vi "Lab0_labview_front_panel.vi"() -> ()   [LabVIEW 2020]
panel:
  in  "Simulation Length":dbl=40.0
  out "Steady state value reached":bool=TRUE
  out "Waveform Chart":dbl(graph)=0.4999988027378587
  out "Current y_n":dbl
  in  "delta t":dbl=0.1
  out "Current Simulation step n":i32
  in  "Stop Simulation":bool
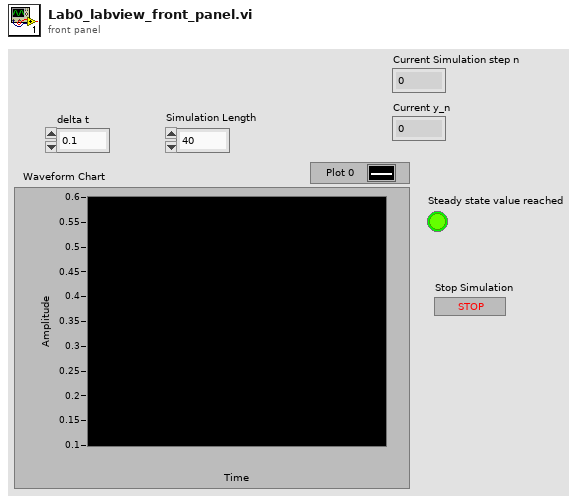
[diagram p1: front panel]
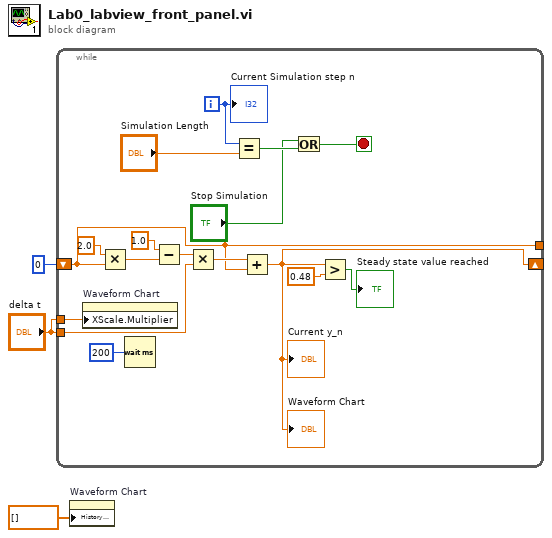
[diagram p0: block diagram]
diagram:
  n1 = while {
    shift-right: [w11] -> _
    shift-left: 0 -> [w10]
    tunnel: "delta t" -> [w15]
    tunnel: [w10] -> _
    tunnel: "delta t" -> [w4]
    i -> [w5]
    stop <- w7 stop-if-true
    n2 = property on="Waveform Chart" class="WFChart (strict)"("XScale.Multiplier"=w4) -> ()  [unwired: 2 in, 2 out]
    n3 = Multiply(x=2.0, y=w10) -> (x*y=w18:dbl)
    n4 = Wait (ms)(milliseconds to wait=u32 200) -> ()  [unwired: 1 out]
    n5 = Subtract(x=1.0, y=w18) -> (x-y=w16:dbl)
    n6 = Multiply(x=w16, y=w15) -> (x*y=w14:dbl)
    n7 = Equal?(x=w5, y="Simulation Length") -> (x = y?=w9:bool)
    n8 = Add(x=w14, y=w10) -> (x+y=w11:dbl)
    "Waveform Chart" <- w11
    "Current y_n" <- w11
    n9 = Or(x="Stop Simulation", y=w9) -> (x .or. y?=w7:bool)
    n10 = Greater?(x=w11, y=0.48 ("x")) -> (0:→"Steady state value reached":bool)
    "Current Simulation step n" <- w5
  }
  n11 = property on="Waveform Chart" class="WFChart (strict)"("History Data"=dbl[] []) -> ()  [unwired: 2 in, 2 out]
